vi "Informacion_A_Canales_Activos.vi"(1 "Canal_Activo_2":bool, 2 "Canal_Activo_1":bool, 3 "Data_Canal_2":dbl, 4 "Data_Canal_1":dbl) -> (0 "Data":dynamicdata(waveform))   [LabVIEW 2023]
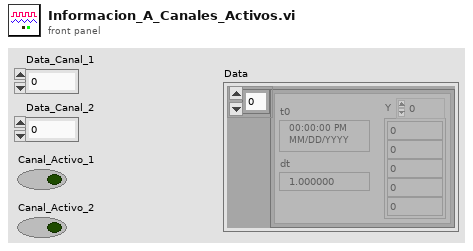
[diagram p1: front panel]
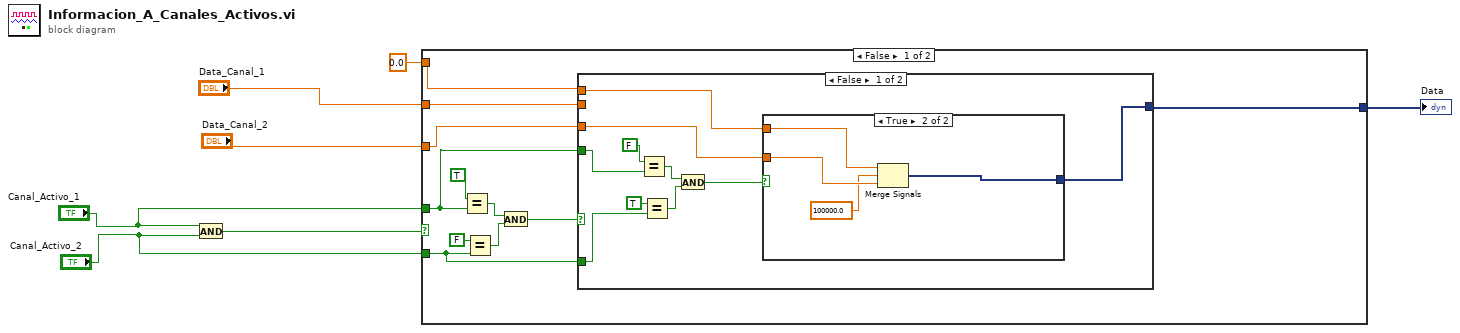
[diagram p0: block diagram]
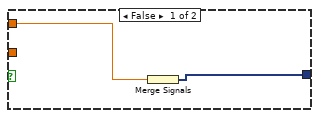
[diagram p2: hidden frame]
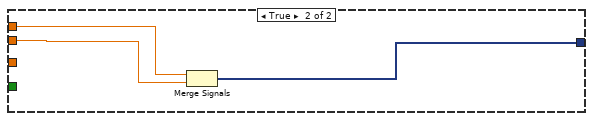
[diagram p3: hidden frame]
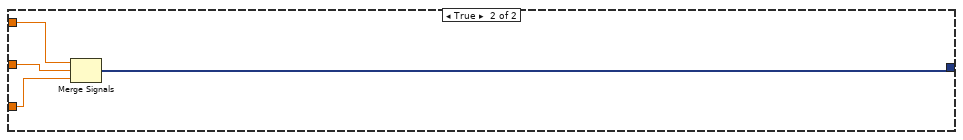
[diagram p4: hidden frame]
diagram:
  n1 = And(x="Canal_Activo_1", y="Canal_Activo_2") -> (x .and. y?=w1:bool)
  n2 = case shown="False" w1 {
    tunnel: 0.0 -> [w13 w41]
    tunnel: [w10 w40] -> w5
    tunnel: "Canal_Activo_2" -> [w9 _]
    tunnel: "Canal_Activo_1" -> [w8 _]
    tunnel: "Data_Canal_2" -> [w11 w38]
    tunnel: "Data_Canal_1" -> [w12 w39]
    frame False {
      n3 = Equal?(x=TRUE, y=w8) -> (x = y?=w15:bool)
      n4 = Equal?(x=FALSE, y=w9) -> (x = y?=w16:bool)
      n5 = And(x=w15, y=w16) -> (x .and. y?=w14:bool)
      n6 = case shown="False" w14 {
        tunnel: w13 -> [w21 w37]
        tunnel: w12 -> [_ w36]
        tunnel: w11 -> [w20 _]
        tunnel: [w19 w35] -> w10
        tunnel: w9 -> [w24 _]
        tunnel: w8 -> [w23 _]
        frame False {
          n7 = Equal?(x=FALSE, y=w23) -> (x = y?=w25:bool)
          n8 = Equal?(x=TRUE, y=w24) -> (x = y?=w26:bool)
          n9 = And(x=w25, y=w26) -> (x .and. y?=w22:bool)
          n10 = case shown="True" w22 {
            tunnel: w21 -> [w30 w32]
            tunnel: w20 -> [_ w34]
            tunnel: [w29 w33] -> w19
            frame False {
              n11 = Merge Signals(w30) -> (w29:dynamicdata)
            }
            frame True {
              n12 = Merge Signals(w32, 100000.0, w34) -> (w33:dynamicdata)
            }
          }
        }
        frame True {
          n13 = Merge Signals(w37, w36) -> (w35:dynamicdata)
        }
      }
    }
    frame True {
      n14 = Merge Signals(w41, w39, w38) -> (w40:dynamicdata)
    }
  }
  "Data" <- w5
